vi "UMLEditor menuUpdates.vi"(0 "menu":refnum<k9>, 1 "menuAction":T1, 2 "item":string, 3 "addfirst(false)":bool, 5 "error in (no error)":errorcluster) -> (19 "error out":errorcluster)   [LabVIEW 2020]
doc: "Gets current diagram values"
uses:
  <resource>/Framework/Providers/Open_GDS/UML/UMLEditor/UMLEditor MenuActionType.ctl
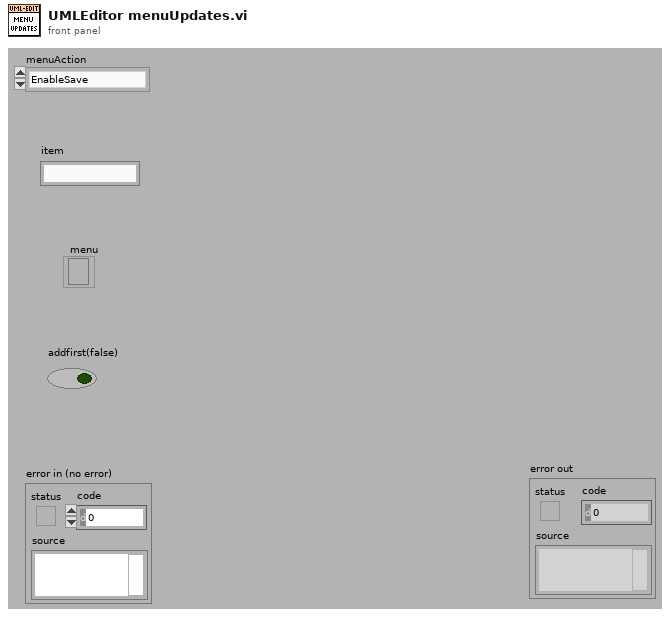
[diagram p1: front panel]
types:
  T1 = typedef "UMLEditor MenuActionType.ctl" = enum16{"EnableSave", "EnablePaste", "DisablePaste", "DiableSave", "AddRecentFile", "disablePropDel", "enablePropDel", "enablePropDisDel", "diasbleClassRel", "enableClassRel", "Class", "State", "Other", "EnableXMI", "DisableXMI"}
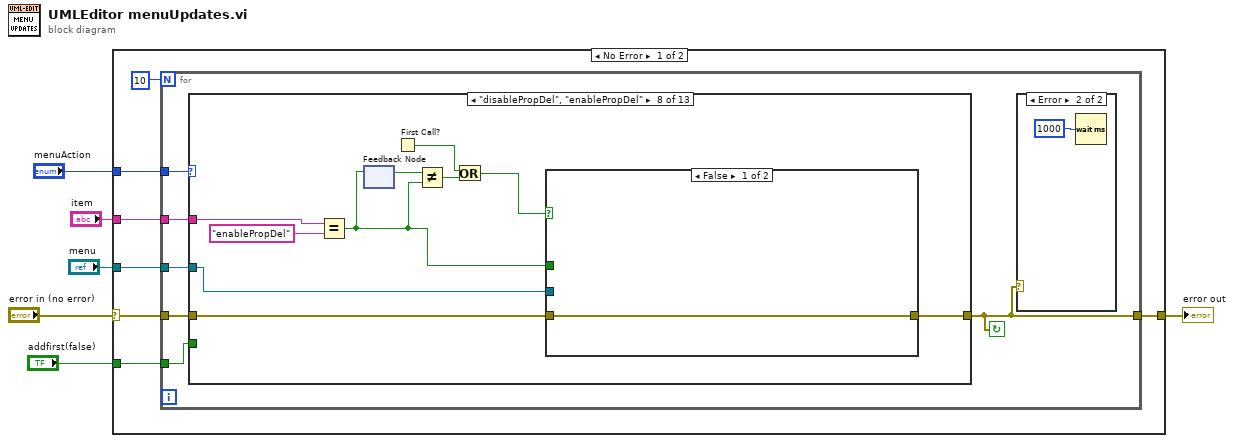
[diagram p0: block diagram]
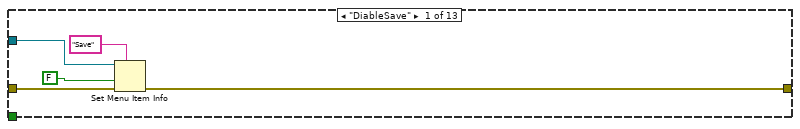
[diagram p3: hidden frame]
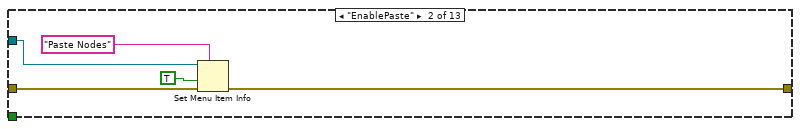
[diagram p4: hidden frame]
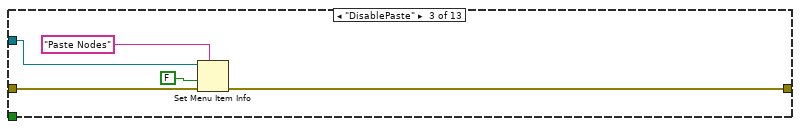
[diagram p5: hidden frame]
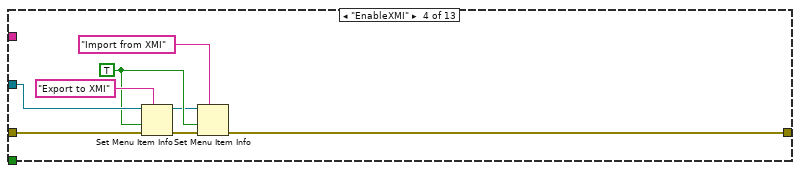
[diagram p6: hidden frame]
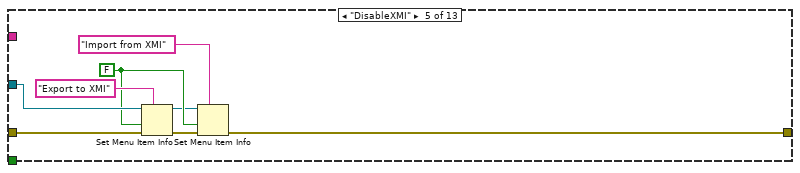
[diagram p7: hidden frame]
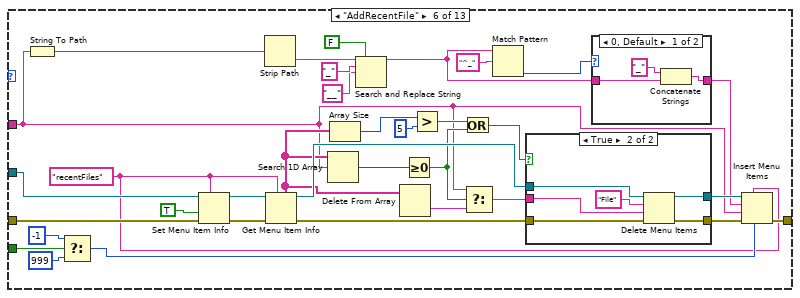
[diagram p8: hidden frame]
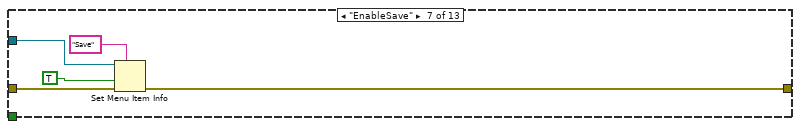
[diagram p11: hidden frame]
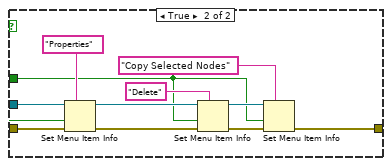
[diagram p12: hidden frame]
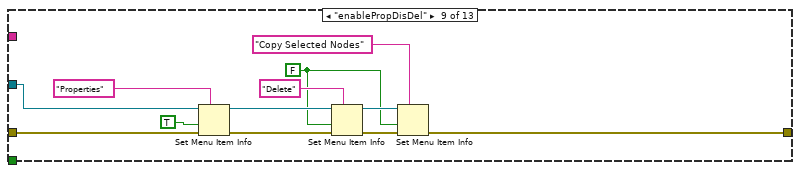
[diagram p13: hidden frame]
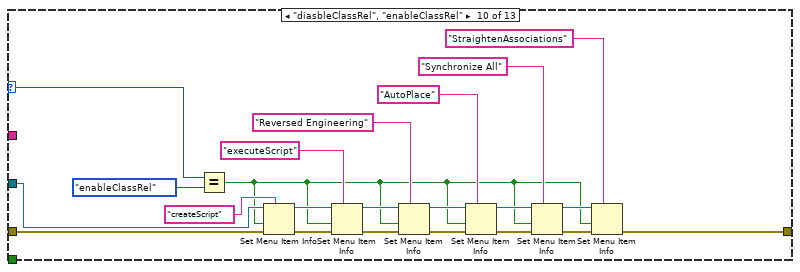
[diagram p14: hidden frame]
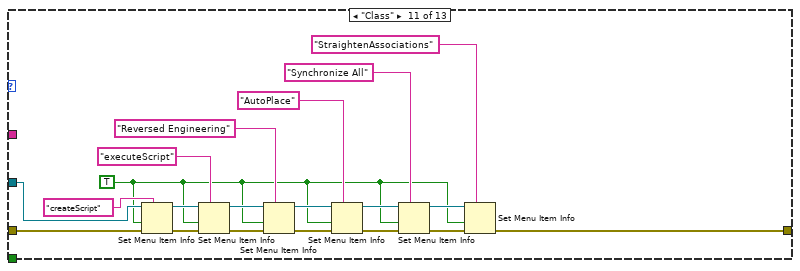
[diagram p15: hidden frame]
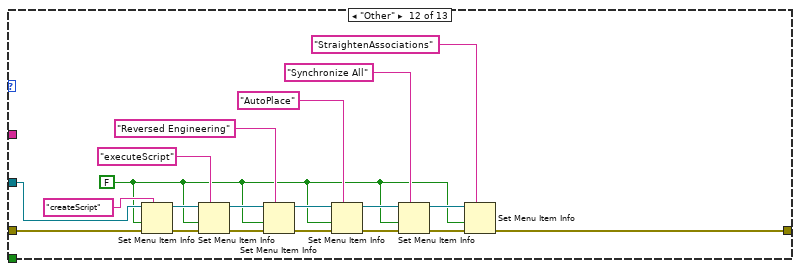
[diagram p16: hidden frame]
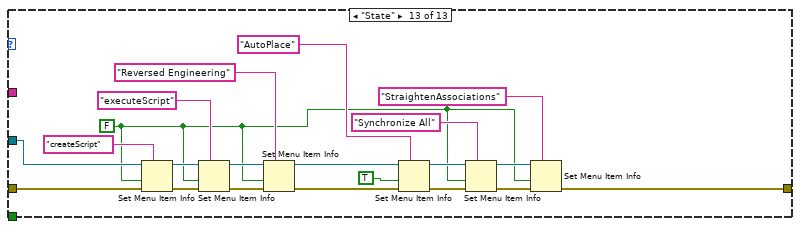
[diagram p17: hidden frame]
diagram:
  n1 = case shown="No Error" "error in (no error)" {
    selector: "error in (no error)" -> [w13 w220]
    tunnel: [w12 w220] -> w5
    tunnel: "menuAction" -> [w11 _]
    tunnel: "item" -> [w10 _]
    tunnel: "addfirst(false)" -> [w9 _]
    tunnel: "menu" -> [w8 _]
    frame No Error {
      n2 = for {
        N: 10 -> [_]
        tunnel: w11 -> [w18]
        tunnel: w10 -> [w17]
        tunnel: w9 -> [w16]
        tunnel: w8 -> [w15]
        tunnel: w13 -> [w19]
        tunnel: [w14] -> w12
        stop <- w14 continue-if-true
        n3 = case shown="\"disablePropDel\", \"enablePropDel\"" w18 {
          selector: w18 -> [_ _ _ _ _ _ _ _ _ w139 _ _ _]
          tunnel: w15 -> [w25 w30 w35 w43 w51 w65 w102 w112 w136 w158 w178 w198 w219]
          tunnel: w19 -> [w24 w29 w34 w42 w50 w63 w101 w111 w135 w157 w177 w197 w218]
          tunnel: [w23 w28 w33 w38 w47 w85 w100 w110 w126 w140 w160 w180 w201] -> w14
          tunnel: w17 -> [_ _ _ _ _ w72 _ w109 _ _ _ _ _]
          tunnel: w16 -> [_ _ _ _ _ w69 _ _ _ _ _ _ _]
          frame "DiableSave" {
            n4 = Set Menu Item Info(7:"Save" ("item tag"), 8:w24, 9:FALSE ("enabled"), 11:w25) -> (0:w23:errorcluster)  [unwired: 4 out]
          }
          frame "EnablePaste" {
            n5 = Set Menu Item Info(7:"Paste Nodes" ("item tag"), 8:w29, 9:TRUE ("enabled"), 11:w30) -> (0:w28:errorcluster)  [unwired: 4 out]
          }
          frame "DisablePaste" {
            n6 = Set Menu Item Info(7:"Paste Nodes" ("item tag"), 8:w34, 9:FALSE ("enabled"), 11:w35) -> (0:w33:errorcluster)  [unwired: 4 out]
          }
          frame "EnableXMI" {
            w37 = TRUE ("enabled")
            n7 = Set Menu Item Info(7:"Export to XMI" ("item tag"), 8:w42, 9:w37, 11:w43) -> (0:w39:errorcluster, 3:w36:refnum<k9>)  [unwired: 3 out]
            n8 = Set Menu Item Info(7:"Import from XMI" ("item tag"), 8:w39, 9:w37, 11:w36) -> (0:w38:errorcluster)  [unwired: 4 out]
          }
          frame "DisableXMI" {
            w45 = FALSE ("enabled")
            n9 = Set Menu Item Info(7:"Export to XMI" ("item tag"), 8:w50, 9:w45, 11:w51) -> (0:w48:errorcluster, 3:w44:refnum<k9>)  [unwired: 3 out]
            n10 = Set Menu Item Info(7:"Import from XMI" ("item tag"), 8:w48, 9:w45, 11:w44) -> (0:w47:errorcluster)  [unwired: 4 out]
          }
          frame "AddRecentFile" {
            w61 = "recentFiles" ("menu tag")
            n11 = String To Path(string=w72) -> (path=w84:path)
            n12 = Select(t=-1, s=w69, f=999) -> (s? t:f=w67:i32)
            n13 = Set Menu Item Info(7:w61, 8:w63, 9:TRUE ("enabled"), 11:w65) -> (0:w62:errorcluster, 3:w64:refnum<k9>)  [unwired: 3 out]
            n14 = Strip Path(path=w84) -> (name=w59:string)  [unwired: 1 out]
            n15 = Get Menu Item Info(7:w61, 8:w62, 11:w64) -> (0:w79:errorcluster, 3:w81:refnum<k9>, 5:w77:string[])  [unwired: 4 out]
            n16 = Search 1D Array(1D array=w77, element=w72) -> (index of element=w74:i32)  [unwired: 1 out]
            n17 = Array Size(array=w77) -> (size(s)=w83:i32)
            n18 = Search and Replace String(replace all?=FALSE ("replace all? (F)"), input string=w59, search string="_", replace string="__" ("replace string (\"\")")) -> (result string=w53:string)  [unwired: 1 in, 6 out]
            n19 = Delete From Array(array=w77) -> (deleted portion=w71:string)  [unwired: 2 in, 1 out]
            n20 = Greater Or Equal To 0?(x=w74) -> (x >= 0?=w73:bool)
            n21 = Greater?(x=w83, y=5) -> (0:w75:bool)
            n22 = Or(x=w75, y=w73) -> (x .or. y?=w76:bool)
            n23 = Select(t=w72, s=w73, f=w71) -> (s? t:f=w70:string)
            n24 = Match Pattern(string=w53, regular expression="^_") -> (offset past match=w54:i32)  [unwired: 4 out]
            n25 = case shown="True" w76 {
              tunnel: w81 -> [w91 w97]
              tunnel: [w91 w96] -> w80
              tunnel: w70 -> [_ w93]
              tunnel: w79 -> [w90 w95]
              tunnel: [w90 w94] -> w78
              frame False {
              }
              frame True {
                n26 = Delete Menu Items(6:w95, 7:w93, 8:"File" ("menu tag"), 9:w97) -> (0:w94:errorcluster, 3:w96:refnum<k9>)
              }
            }
            n27 = case shown="0, Default" w54 {
              tunnel: w53 -> [w88 w89]
              tunnel: [w87 w89] -> w52
              frame 0, Default {
                n28 = Concatenate Strings("_" ("search string"), w88) -> (w87:string)
              }
              frame -1 {
              }
            }
            n29 = Insert Menu Items(4:w67, 5:w61, 6:w78, 7:w72, 8:w52, 9:w80) -> (0:w85:errorcluster)  [unwired: 2 out]
          }
          frame "EnableSave" {
            n30 = Set Menu Item Info(7:"Save" ("item tag"), 8:w101, 9:TRUE ("enabled"), 11:w102) -> (0:w100:errorcluster)  [unwired: 4 out]
          }
          frame "disablePropDel", "enablePropDel" {
            n31 = Equal?(x=w109, y="enablePropDel") -> (x = y?=w106:bool)
            n32 = feedback-in #1(w106) -> ()
            n33 = feedback #1() -> (w107:bool)  [unwired: 1 in]
            n34 = First Call?() -> (First Call?: T/F=w104:bool)
            n35 = Not Equal?(x=w107, y=w106) -> (x != y?=w105:bool)
            n36 = Or(x=w104, y=w105) -> (x .or. y?=w103:bool)
            n37 = case shown="False" w103 {
              tunnel: w112 -> [_ w124]
              tunnel: w111 -> [w113 w123]
              tunnel: [w113 w116] -> w110
              tunnel: w106 -> [_ w114]
              frame False {
              }
              frame True {
                n38 = Set Menu Item Info(7:"Properties" ("item tag"), 8:w123, 9:w114, 11:w124) -> (0:w119:errorcluster, 3:w121:refnum<k9>)  [unwired: 3 out]
                n39 = Set Menu Item Info(7:"Delete" ("item tag"), 8:w119, 9:w114, 11:w121) -> (0:w118:errorcluster, 3:w117:refnum<k9>)  [unwired: 3 out]
                n40 = Set Menu Item Info(7:"Copy Selected Nodes" ("item tag"), 8:w118, 9:w114, 11:w117) -> (0:w116:errorcluster)  [unwired: 4 out]
              }
            }
          }
          frame "enablePropDisDel" {
            w125 = FALSE ("enabled")
            n41 = Set Menu Item Info(7:"Properties" ("item tag"), 8:w135, 9:TRUE ("enabled"), 11:w136) -> (0:w130:errorcluster, 3:w133:refnum<k9>)  [unwired: 3 out]
            n42 = Set Menu Item Info(7:"Delete" ("item tag"), 8:w130, 9:w125, 11:w133) -> (0:w128:errorcluster, 3:w127:refnum<k9>)  [unwired: 3 out]
            n43 = Set Menu Item Info(7:"Copy Selected Nodes" ("item tag"), 8:w128, 9:w125, 11:w127) -> (0:w126:errorcluster)  [unwired: 4 out]
          }
          frame "diasbleClassRel", "enableClassRel" {
            n44 = Equal?(x=w139, y=UMLEditor_MenuActionType."enableClassRel") -> (x = y?=w137:bool)
            n45 = Set Menu Item Info(7:"createScript" ("item tag"), 8:w157, 9:w137, 11:w158) -> (0:w153:errorcluster, 3:w155:refnum<k9>)  [unwired: 3 out]
            n46 = Set Menu Item Info(7:"executeScript" ("item tag"), 8:w153, 9:w137, 11:w155) -> (0:w149:errorcluster, 3:w152:refnum<k9>)  [unwired: 3 out]
            n47 = Set Menu Item Info(7:"Reversed Engineering" ("item tag"), 8:w149, 9:w137, 11:w152) -> (0:w151:errorcluster, 3:w150:refnum<k9>)  [unwired: 3 out]
            n48 = Set Menu Item Info(7:"AutoPlace" ("item tag"), 8:w151, 9:w137, 11:w150) -> (0:w145:errorcluster, 3:w144:refnum<k9>)  [unwired: 3 out]
            n49 = Set Menu Item Info(7:"Synchronize All" ("item tag"), 8:w145, 9:w137, 11:w144) -> (0:w141:errorcluster, 3:w142:refnum<k9>)  [unwired: 3 out]
            n50 = Set Menu Item Info(7:"StraightenAssociations" ("item tag"), 8:w141, 9:w137, 11:w142) -> (0:w140:errorcluster)  [unwired: 4 out]
          }
          frame "Class" {
            w159 = TRUE ("enabled")
            n51 = Set Menu Item Info(7:"createScript" ("item tag"), 8:w177, 9:w159, 11:w178) -> (0:w173:errorcluster, 3:w175:refnum<k9>)  [unwired: 3 out]
            n52 = Set Menu Item Info(7:"executeScript" ("item tag"), 8:w173, 9:w159, 11:w175) -> (0:w169:errorcluster, 3:w172:refnum<k9>)  [unwired: 3 out]
            n53 = Set Menu Item Info(7:"Reversed Engineering" ("item tag"), 8:w169, 9:w159, 11:w172) -> (0:w171:errorcluster, 3:w170:refnum<k9>)  [unwired: 3 out]
            n54 = Set Menu Item Info(7:"AutoPlace" ("item tag"), 8:w171, 9:w159, 11:w170) -> (0:w165:errorcluster, 3:w164:refnum<k9>)  [unwired: 3 out]
            n55 = Set Menu Item Info(7:"Synchronize All" ("item tag"), 8:w165, 9:w159, 11:w164) -> (0:w161:errorcluster, 3:w162:refnum<k9>)  [unwired: 3 out]
            n56 = Set Menu Item Info(7:"StraightenAssociations" ("item tag"), 8:w161, 9:w159, 11:w162) -> (0:w160:errorcluster)  [unwired: 4 out]
          }
          frame "Other" {
            w179 = FALSE ("enabled")
            n57 = Set Menu Item Info(7:"createScript" ("item tag"), 8:w197, 9:w179, 11:w198) -> (0:w193:errorcluster, 3:w195:refnum<k9>)  [unwired: 3 out]
            n58 = Set Menu Item Info(7:"executeScript" ("item tag"), 8:w193, 9:w179, 11:w195) -> (0:w189:errorcluster, 3:w192:refnum<k9>)  [unwired: 3 out]
            n59 = Set Menu Item Info(7:"Reversed Engineering" ("item tag"), 8:w189, 9:w179, 11:w192) -> (0:w191:errorcluster, 3:w190:refnum<k9>)  [unwired: 3 out]
            n60 = Set Menu Item Info(7:"AutoPlace" ("item tag"), 8:w191, 9:w179, 11:w190) -> (0:w185:errorcluster, 3:w184:refnum<k9>)  [unwired: 3 out]
            n61 = Set Menu Item Info(7:"Synchronize All" ("item tag"), 8:w185, 9:w179, 11:w184) -> (0:w181:errorcluster, 3:w182:refnum<k9>)  [unwired: 3 out]
            n62 = Set Menu Item Info(7:"StraightenAssociations" ("item tag"), 8:w181, 9:w179, 11:w182) -> (0:w180:errorcluster)  [unwired: 4 out]
          }
          frame "State" {
            w200 = FALSE ("enabled")
            n63 = Set Menu Item Info(7:"createScript" ("item tag"), 8:w218, 9:w200, 11:w219) -> (0:w214:errorcluster, 3:w216:refnum<k9>)  [unwired: 3 out]
            n64 = Set Menu Item Info(7:"executeScript" ("item tag"), 8:w214, 9:w200, 11:w216) -> (0:w210:errorcluster, 3:w213:refnum<k9>)  [unwired: 3 out]
            n65 = Set Menu Item Info(7:"Reversed Engineering" ("item tag"), 8:w210, 9:w200, 11:w213) -> (0:w212:errorcluster, 3:w211:refnum<k9>)  [unwired: 3 out]
            n66 = Set Menu Item Info(7:"AutoPlace" ("item tag"), 8:w212, 9:TRUE ("enabled"), 11:w211) -> (0:w206:errorcluster, 3:w205:refnum<k9>)  [unwired: 3 out]
            n67 = Set Menu Item Info(7:"Synchronize All" ("item tag"), 8:w206, 9:w200, 11:w205) -> (0:w202:errorcluster, 3:w203:refnum<k9>)  [unwired: 3 out]
            n68 = Set Menu Item Info(7:"StraightenAssociations" ("item tag"), 8:w202, 9:w200, 11:w203) -> (0:w201:errorcluster)  [unwired: 4 out]
          }
        }
        n69 = case shown="Error" w14 {
          frame No Error {
          }
          frame Error {
            n70 = Wait (ms)(milliseconds to wait=u32 1000) -> ()  [unwired: 1 out]
          }
        }
      }
    }
    frame Error {
    }
  }
  "error out" <- w5
